vi "Main.vi"() -> ()   [LabVIEW 2023]
uses:
  Application_class/Application.lvclass
  <vilib>/Utility/error.llb/Error Cluster From Error Code.vi
  <vilib>/ErrorRing/Error Ring.xnode
  AFG3022B_class/AFG3022B.lvclass
  CetoniPump_class/CetoniPump.lvclass
  AD2_SDK_class/AD2_SDK.lvclass
  TBS2000Series_class/TBS2000Series.lvclass
  AD2_WFG_SDK_class/AD2TriggerSources.ctl
  AD2_DO_SDK_class/DOTrigger.ctl
  AD2_DO_SDK_class/AD2_DO_SDK.lvclass
  AD2_DO_SDK_class/DOCustomData.ctl
  AD2_DO_SDK_class/DOConfigureCustomData.ctl
  TC0608_class/TC0608.lvclass
  SaveData_class/SaveData.lvclass
  AD2_MSO_SDK_class/AD2TriggerSources.ctl
  AD2_MSO_SDK_class/AD2_MSO_SDK.lvclass
  AD2_MSO_SDK_class/MSORangeCh.ctl
  AD2_MSO_SDK_class/MSOConfig.ctl
panel:
  out "Pump Status":T1(array[cluster])
  in  "Tab Control":T2(tab)=enum."Debug"
  in  "Peltier Controller":bool
  in  "Oscilloscope":bool
  in  "Function Generator":bool
  in  "Cetoni Pump":bool
  in  "Analog Discovery":bool
  in  "Init":bool
  in  "Function Generator":refnum<visa-resource-name>
  in  "Oscilloscope":refnum<visa-resource-name>
  in  "Peltier VISA resource name":refnum<visa-resource-name>
  in  "Device Configuration Folder":string="C:\\Users\\Public\\Documents\\QmixElements\\Projects\\default_project\\Configurations\\sinle"
  in  "Read Peltier":bool
  out "temperature (C)":dbl
  in  "Amplitude Step Number":dbl
  in  "End Amplitude":dbl
  in  "Start Amplitude":dbl
  in  "Frequency Step Size":dbl
  in  "Frequency Step Number":dbl
  in  "Resonance Frequency":dbl
  in  "Voltage Series":bool
  in  "Manual Voltage":bool
  in  "Frequency Series":bool
  in  "Manual Frequency":bool
  in  "Frequency (1000 Hz)":dbl=1000.0
  in  "Amplitude (1 Vpp)":dbl=1.0
  in  "STOP ALL PUMPS!":bool
  in  "GoToLevelSettings":T3
  in  "Go To Level":bool
  in  "Refill":bool
  in  "Index":i32
  in  "Empty":bool
  in  "Read Status":bool
  in  "Configure Syringe":bool
  in  "index configure syringe":i32
  in  "SyringeSettings":T4={"Maximum Piston Stroke (mm)"=100.0, "Inner Diameter (mm)"=12.0}
  in  "Reference Move":bool
  in  "Take Images":bool
  in  "Image  Aquisition":T5={"Minimum Time between frames(s)"=10.0, "Number of Frames"=0} {"Minimum Time between frames(s)" min=0.005}
  in  "Configure MSO":bool
  in  "MSO":T6={"Timing"={"Enable"=TRUE, "Samples In"=100000.0, "Sample Rate"=1250000.0, "Mode"=enum."Single Sample"}, "Trigger"={"Hysteresis"=0.0, "Trigger Level"=0.0, "Trigger Condition"=0, "Trigger Type"=0, "Trigger Channel"=0, "secTimeout"=1.0, "TrigrSrc"=enum."trigrsrcNone"}, "Range Ch1"={"idxChannel"=0, "voltOffset"=0.0, "VoltsRange"=50}, "Range Ch 2"={"idxChannel"=1, "voltOffset"=0.0, "VoltsRange"=50}} {"Range Ch 2"."VoltsRange" items=["High 50V"=50, "Low5V"=5]; "Range Ch1"."VoltsRange" items=["High 50V"=50, "Low5V"=5]; "Trigger"."Trigger Channel" items=["Channel 1"=0, "Channel 2"=1, "Both"=-1]; "Trigger"."Trigger Type" items=["Edge", "Pulse", "Transition"]; "Trigger"."Trigger Condition" items=["Rising", "Falling"]}
  in  "Read MSO":bool
  out "Waveform Graph":waveform(dbl)[](graph)
  in  "Oscilloscope":T9={"Source Main"=2, "Source Probe"=1, "Source Prefocus"=2} {"Source Prefocus" items=["Math", "Channel 1", "Channel 2", "Channel 3", "Channel 4"]; "Source Probe" items=["Math", "Channel 1", "Channel 2", "Channel 3", "Channel 4"]; "Source Main" items=["Math", "Channel 1", "Channel 2", "Channel 3", "Channel 4"]}
  in  "Start Experiment":bool
  out "Temperatur (C)":dbl
  in  "Experiment Settings":T10={"Frequencies (MHz)"=[], "Camera Settings"={"Minimum Time between\n frames(s)"=10.0, "Number of Frames"=0}, "Flowrates (ul/min)"=[], "Voltages (V)"=[]} {"Camera Settings"."Minimum Time between\n frames(s)" min=0.005}
  in  "SaveFolder":path
  out "Oscilloscope Results":T11 {"Probe Current" format="%.2p"; "Phase Angle" format="%.2p"; "Main Freq" format="%.2p"; "Main Volt" format="%.2p"; "Prefocus Freq" format="%.2p"; "Prefocus Volt" format="%.2p"}
  out "LOG":string
  in  "Time To wait":dbl
  in  "Wait":bool
  in  "index":i32
  in  "refill below level":dbl
  in  "Timeout Refill":dbl=20.0 caption="Time Target (s)"
  in  "Check Level and Refill":bool
  in  "Inject Error<Replace Me>":bool
  in  "Trigg AD2":bool
  in  "Configure DO":bool
  in  "?":T12={"DO Trigger"={"secRun(0=Cont)"=0.0, "secWait"=0.0, "cRepeat(0=inf)"=0, "Repeat Trigger"=TRUE, "TrigrSrc"=enum."trigsrcPC"}, "CustomData"=[{"Data"=[FALSE, TRUE, FALSE, FALSE, FALSE, FALSE, FALSE, FALSE, FALSE, FALSE, FALSE, FALSE, FALSE, FALSE, FALSE, FALSE, FALSE, FALSE, FALSE, FALSE, FALSE, FALSE], "Freq"=1000.0, "#Bits"=100, "Enable"=TRUE, "IdleState"=0}, {"Data"=[], "Freq"=0.0, "#Bits"=0, "Enable"=FALSE, "IdleState"=0}, {"Data"=[], "Freq"=0.0, "#Bits"=0, "Enable"=FALSE, "IdleState"=0}, {"Data"=[], "Freq"=0.0, "#Bits"=0, "Enable"=FALSE, "IdleState"=0}, {"Data"=[], "Freq"=0.0, "#Bits"=0, "Enable"=FALSE, "IdleState"=0}, {"Data"=[], "Freq"=0.0, "#Bits"=0, "Enable"=FALSE, "IdleState"=0}, {"Data"=[], "Freq"=0.0, "#Bits"=0, "Enable"=FALSE, "IdleState"=0}, {"Data"=[], "Freq"=0.0, "#Bits"=0, "Enable"=FALSE, "IdleState"=0}, {"Data"=[], "Freq"=0.0, "#Bits"=0, "Enable"=FALSE, "IdleState"=0}, {"Data"=[], "Freq"=0.0, "#Bits"=0, "Enable"=FALSE, "IdleState"=0}, {"Data"=[], "Freq"=0.0, "#Bits"=0, "Enable"=FALSE, "IdleState"=0}, {"Data"=[], "Freq"=0.0, "#Bits"=0, "Enable"=FALSE, "IdleState"=0}, {"Data"=[], "Freq"=0.0, "#Bits"=0, "Enable"=FALSE, "IdleState"=0}, {"Data"=[FALSE, FALSE, FALSE, FALSE, FALSE, FALSE, FALSE, FALSE, FALSE, FALSE, FALSE, FALSE, FALSE, FALSE, FALSE, FALSE, FALSE, FALSE, FALSE, FALSE, FALSE, FALSE, FALSE], "Freq"=0.0, "#Bits"=0, "Enable"=FALSE, "IdleState"=0}, {"Data"=[FALSE, FALSE, FALSE, FALSE, FALSE, FALSE, FALSE, FALSE, FALSE, FALSE, FALSE, FALSE, FALSE, FALSE, FALSE, FALSE, FALSE, FALSE, FALSE, FALSE, FALSE, FALSE, FALSE], "Freq"=0.0, "#Bits"=0, "Enable"=FALSE, "IdleState"=0}]}
  in  "ABORT":bool
  out "Status":string="Program Started\nPlease connect to instruments"
  out "error out":errorcluster
  in  "Exit":bool
  # "Include connection of Pump, Camera and Multimeter as well. Have some feedback (LED) if connected."
  # "Select Instruments to Initialize"
  # "FREQUENCY"
  # "VOLTAGE"
  # "There needs to be some build-in control to reverse the pump (refilling it and mixing the particles at the same time) \nafter each completed Frequency Series"
  # "Makse sure to set minimim time large enough, otherwise camera will ignore triggers and we skip frames\nSince we are not running with SDK we cannot know if Images are taken or not"
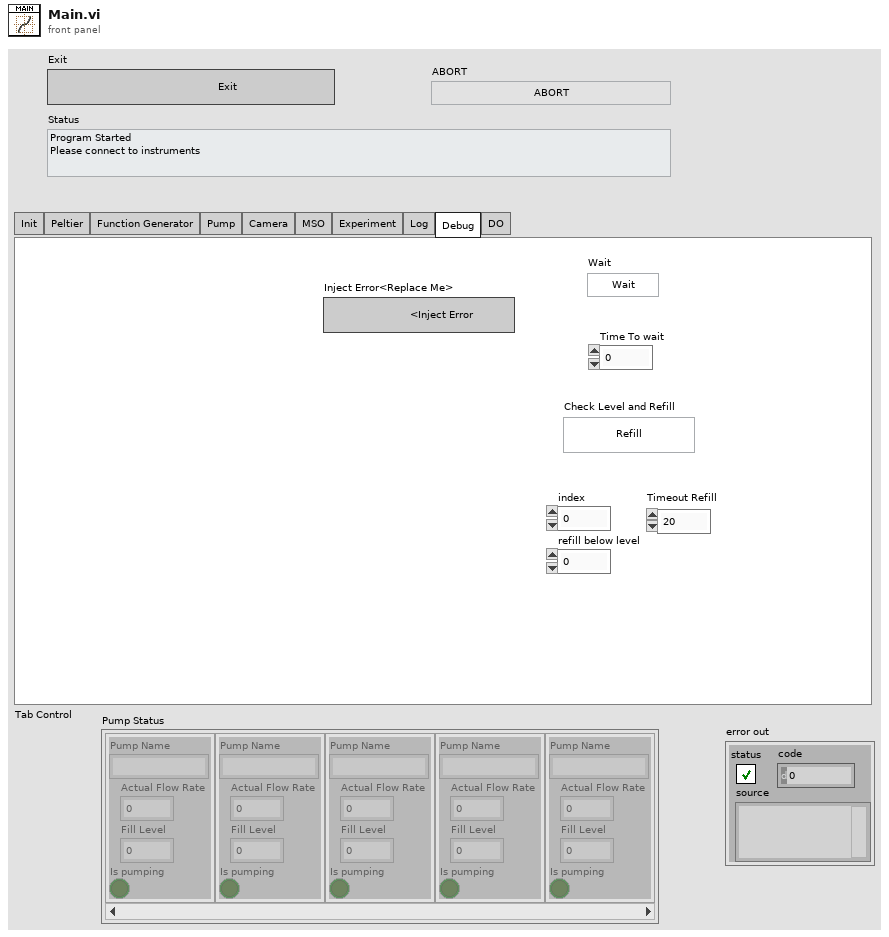
[diagram p1: front panel]
types:
  T1 = cluster{"Pump Name":string, "Actual Flow Rate":dbl, "Fill Level":dbl, "Is pumping":bool}[]
  T2 = enum32{"Init", "Peltier", "Function Generator", "Pump", "Camera", "MSO", "Experiment", "Log", "Debug", "DO"}
  T3 = cluster{"index":i32, "Level(ml)":dbl, "Flow":dbl}
  T4 = cluster{"Maximum Piston Stroke (mm)":dbl, "Inner Diameter (mm)":dbl}
  T5 = cluster{"Minimum Time between frames(s)":dbl, "Number of Frames":i32}
  T6 = typedef "AD2_MSO_SDK.lvclass/MSOConfig.ctl" = cluster{"Timing":cluster{"Enable":bool, "Samples In":dbl, "Sample Rate":dbl, "Mode":enum16{"Single Sample", "Scanshift", "Multiple Samples", "Scan Screen"}}, "Trigger":cluster{"Hysteresis":dbl, "Trigger Level":dbl, "Trigger Condition":i32, "Trigger Type":i32, "Trigger Channel":i32, "secTimeout":dbl, "TrigrSrc":T7}, "Range Ch1":T8, "Range Ch 2":T8}
  T7 = typedef "AD2_MSO_SDK.lvclass/AD2TriggerSources.ctl" = enum8{"trigrsrcNone", "trigsrcPC", "trigsrcDetectorAnalogIn", "trigsrcDetectorDigitalIn", "trigsrcAnalogIn", "trigsrcDigitalIn", "trigsrcDigitalOut", "trigsrcAnalogOut1", "trigsrcAnalogOut2", "trigsrcAnalogOut3", "trigsrcAnalogOut4", "trigsrcExternal1", "trigsrcExternal2", "trigsrcExternal3", "trigsrcExternal4", ""}
  T8 = typedef "AD2_MSO_SDK.lvclass/MSORangeCh.ctl" = cluster{"idxChannel":i32, "voltOffset":dbl, "VoltsRange":u16}
  T9 = cluster{"Source Main":i32, "Source Probe":i32, "Source Prefocus":i32}
  T10 = cluster{"Frequencies (MHz)":dbl[], "Camera Settings":cluster{"Minimum Time between\n frames(s)":dbl, "Number of Frames":i32}, "Flowrates (ul/min)":dbl[], "Voltages (V)":dbl[]}
  T11 = cluster{"Prefocus":cluster{"Initial X":dbl, "X Increment":dbl, "Waveform Array":dbl[]}, "Prefocus Volt":dbl, "Prefocus Freq":dbl, "Main":cluster{"Initial X":dbl, "X Increment":dbl, "Waveform Array":dbl[]}, "Main Volt":dbl, "Main Freq":dbl, "Phase Angle":dbl, "Probe Current":dbl, "Power (Watt)":dbl}
  T12 = typedef "DOConfigureCustomData.ctl" = cluster{"DO Trigger":T13, "CustomData":T15}
  T13 = typedef "AD2_DO_SDK.lvclass/DOTrigger.ctl" = cluster{"secRun(0=Cont)":dbl, "secWait":dbl, "cRepeat(0=inf)":i32, "Repeat Trigger":bool, "TrigrSrc":T14}
  T14 = typedef "AD2_SDK.lvclass/AD2TriggerSources.ctl" = enum8{"trigrsrcNone", "trigsrcPC", "trigsrcDetectorAnalogIn", "trigsrcDetectorDigitalIn", "trigsrcAnalogIn", "trigsrcDigitalIn", "trigsrcDigitalOut", "trigsrcAnalogOut1", "trigsrcAnalogOut2", "trigsrcAnalogOut3", "trigsrcAnalogOut4", "trigsrcExternal1", "trigsrcExternal2", "trigsrcExternal3", "trigsrcExternal4", ""}
  T15 = typedef "AD2_DO_SDK.lvclass/DOCustomData.ctl" = cluster{"Data":bool[], "Freq":dbl, "#Bits":u32, "Enable":bool, "IdleState":u16}[]
  T16 = cluster{"Minimum Time between frames":dbl, "Number of Frames":i32}
  T17 = cluster{"Pump Handle":i64, "Pump Name":string, "Maximum Volume":dbl, "Maximum Flow Rate":dbl, "Flow Rate":dbl, "Target Level":dbl, "Valve Handle":i64, "Has Valve?":bool, "Actual valve position":i32}[]
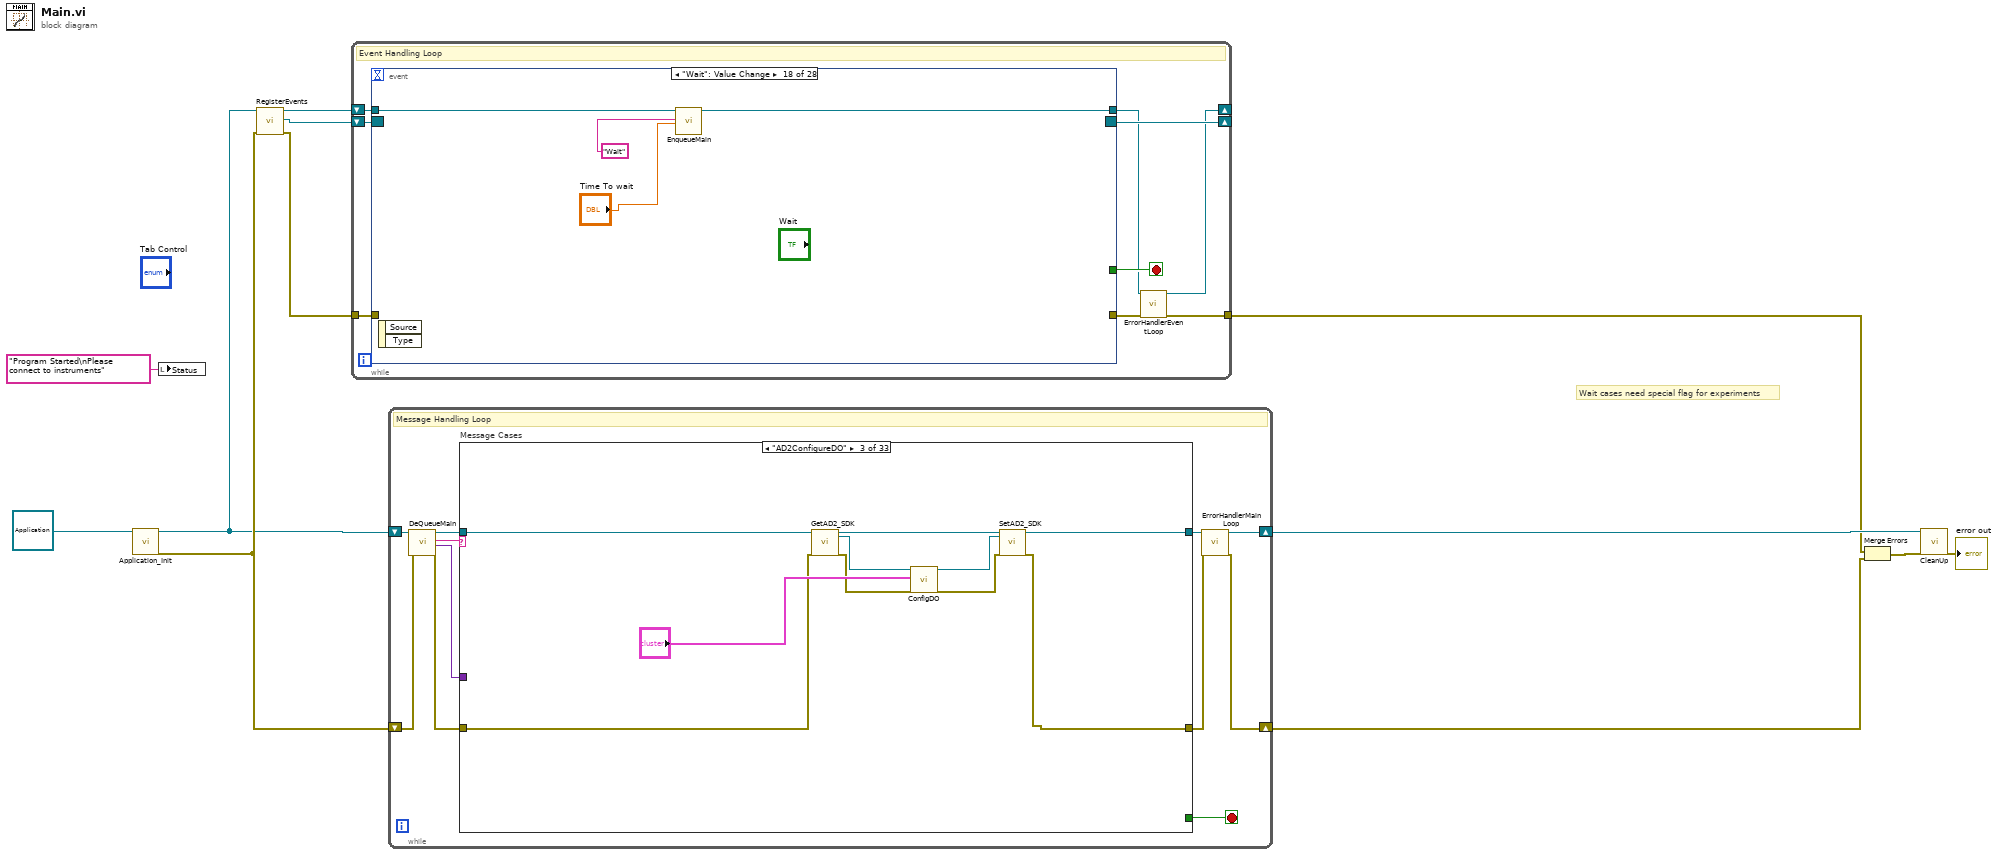
[diagram p0: block diagram]
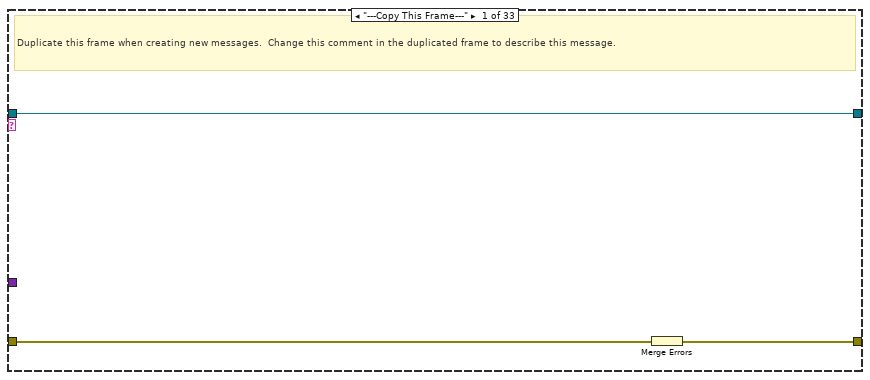
[diagram p2: hidden frame]
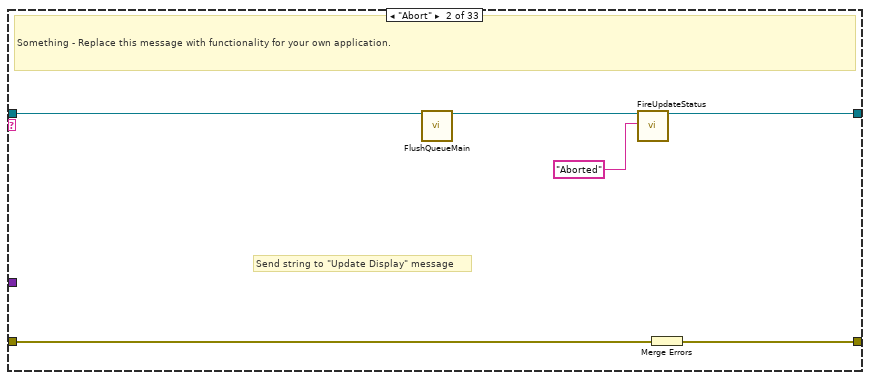
[diagram p3: hidden frame]
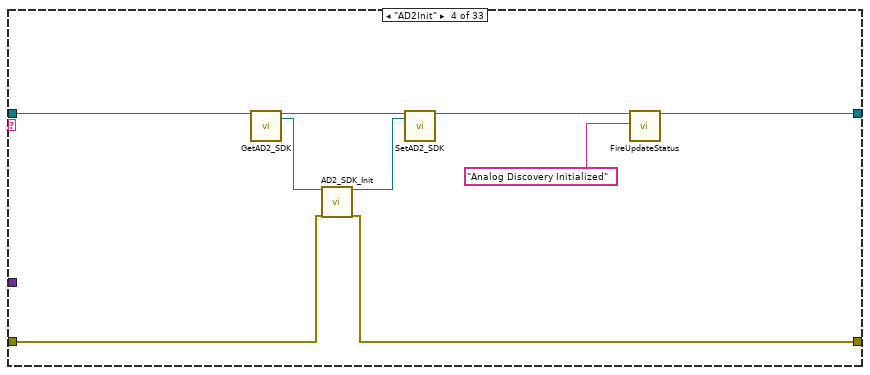
[diagram p4: hidden frame]
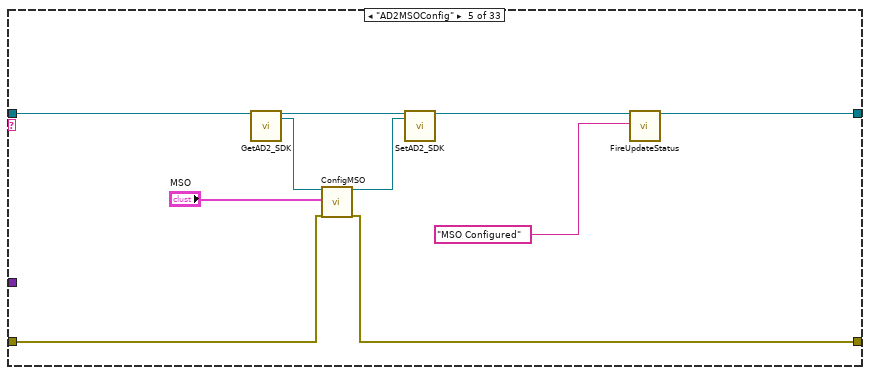
[diagram p5: hidden frame]
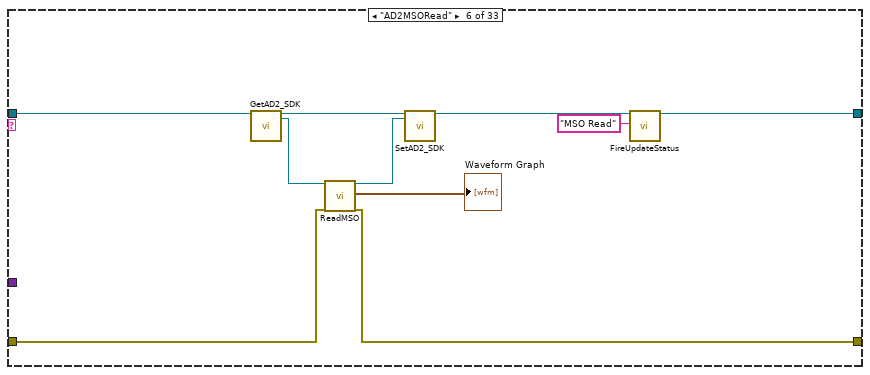
[diagram p6: hidden frame]
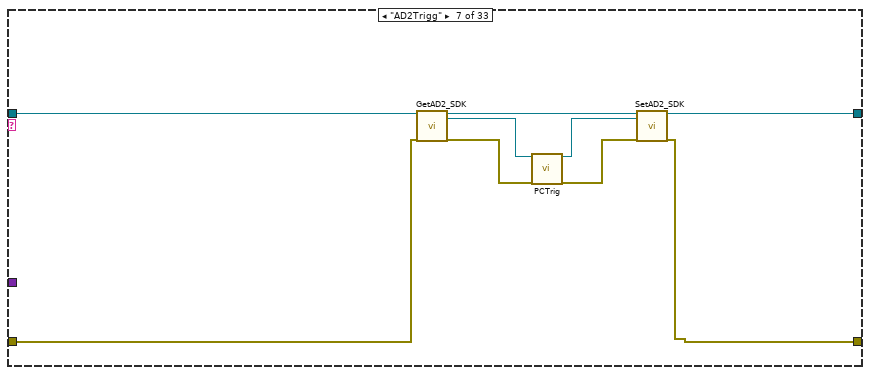
[diagram p7: hidden frame]
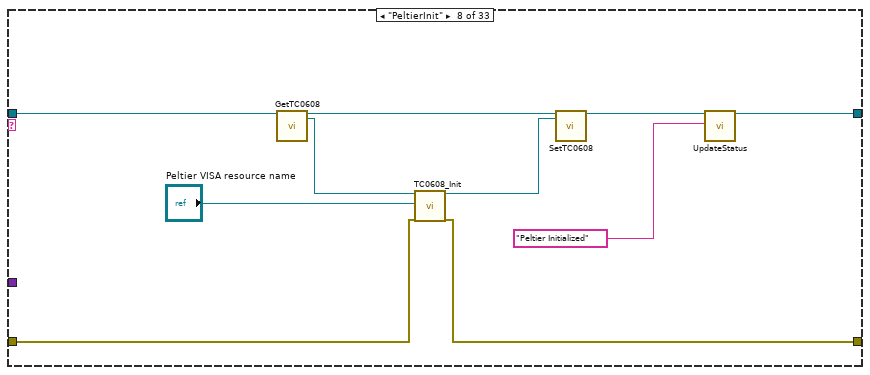
[diagram p8: hidden frame]
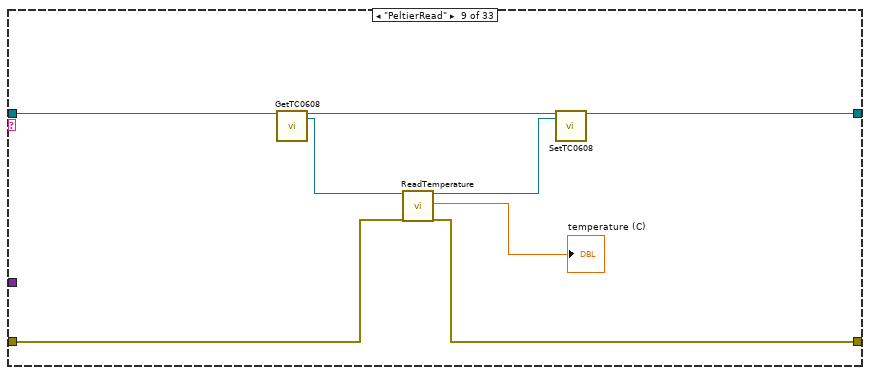
[diagram p9: hidden frame]
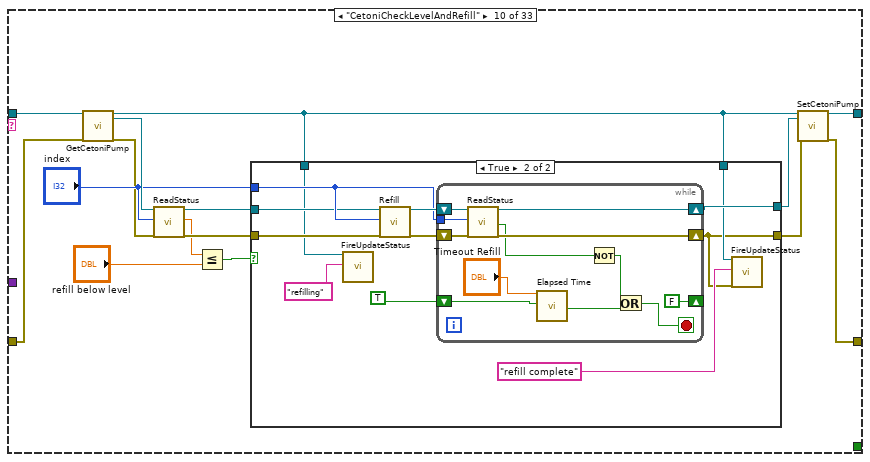
[diagram p10: hidden frame]
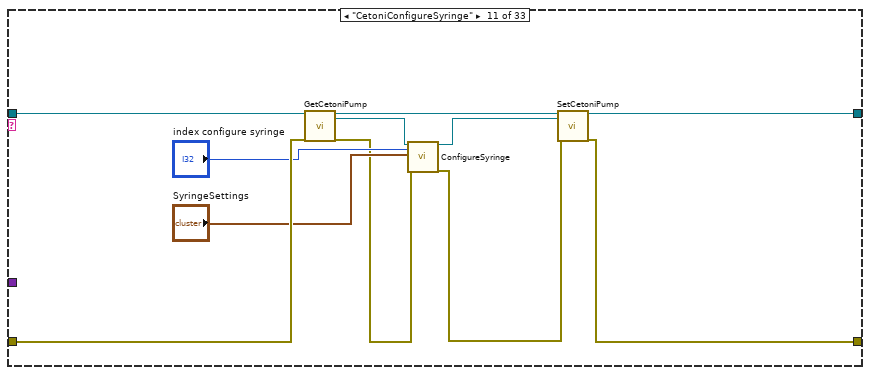
[diagram p12: hidden frame]
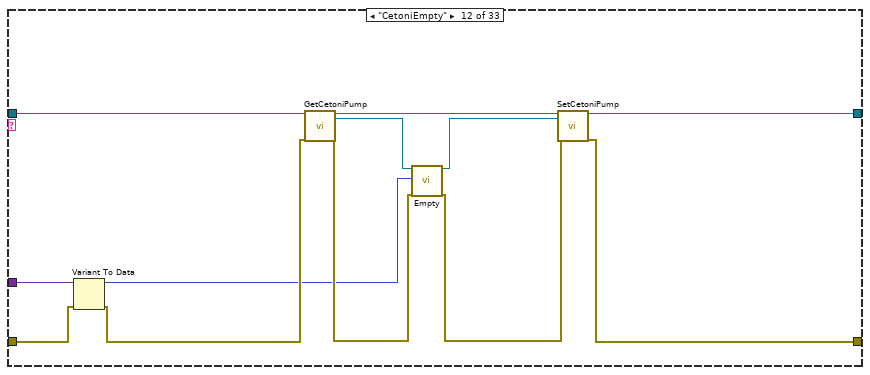
[diagram p13: hidden frame]
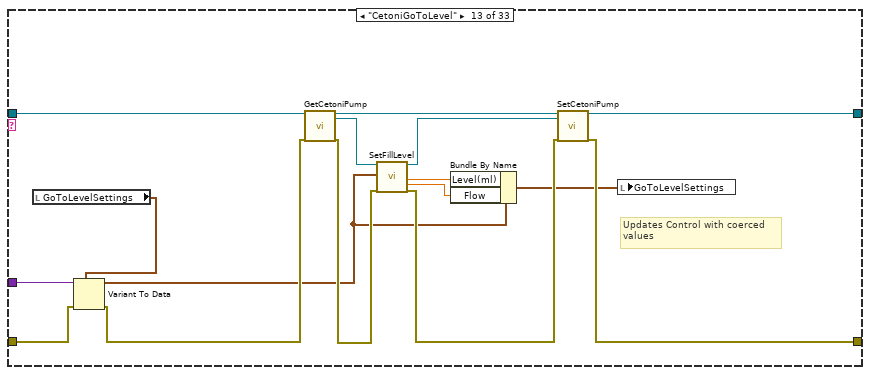
[diagram p14: hidden frame]
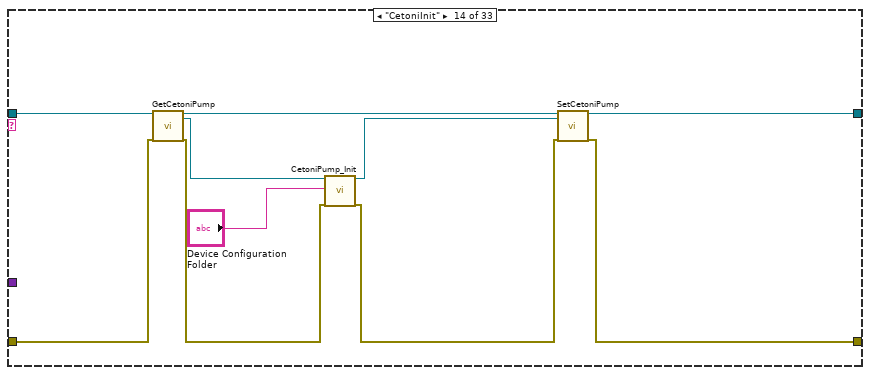
[diagram p15: hidden frame]
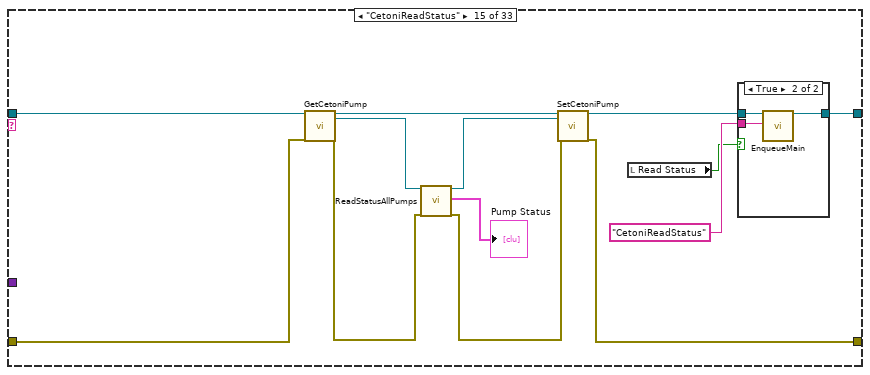
[diagram p16: hidden frame]
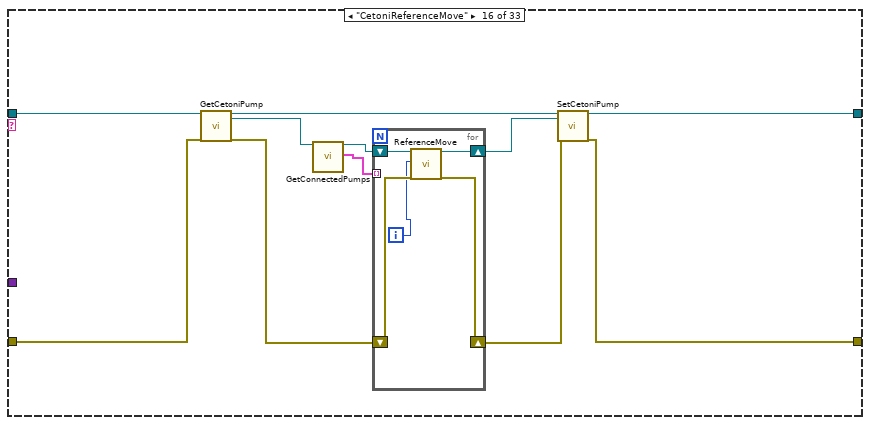
[diagram p18: hidden frame]
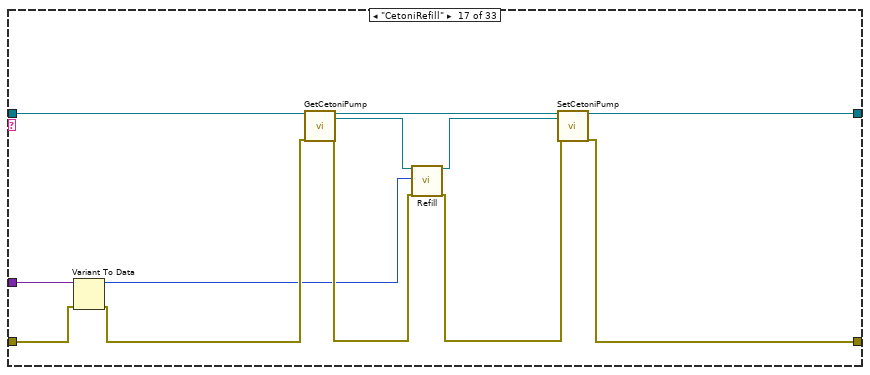
[diagram p19: hidden frame]
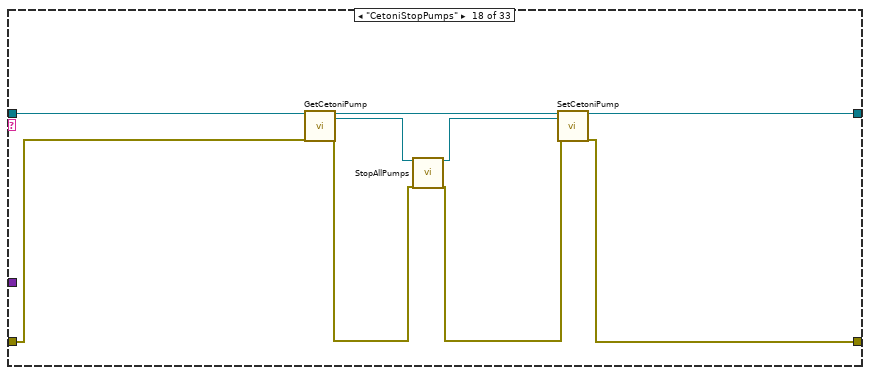
[diagram p20: hidden frame]
diagram:
  # "Wait cases need special flag for experiments"
  n1 = call "Application_Init.vi"("object in"=refnum<class "Application.lvclass"> refnum ("Application")) -> ("object out"=w2:refnum<class "Application.lvclass">, "error out"=w8:errorcluster)  [unwired: 17 in]
  n2 = local write "Status"("Program Started\nPlease connect to instruments" ("Status")) -> ()
  n3 = call-dynamic "RegisterEvents.vi"("object in"=w2, "error in (no error)"=w8) -> ("object out"=w10:refnum<class "Application.lvclass">, "Event Registration Refnum"=w11:refnum<event-registration>, "error out"=w9:errorcluster)  [unwired: 15 in]
  n4 = while {
    shift-right: [w20] -> _
    shift-left: w11 -> [w21]
    tunnel: [w15] -> w5
    shift-right: [w13] -> _
    shift-left: w10 -> [w18]
    tunnel: w9 -> [w17]
    stop <- w19 stop-if-true
    # "Event Handling Loop"
    n5 = event shown="[17] \"Wait\": Value Change" {
      selector: w21 -> [_ _ _ _ _ _ _ _ _ _ _ _ _ _ _ _ _ _ _ _ _ _ _ _ _ _ _ _]
      dyn-events: [_ _ _ _ _ _ _ _ _ _ _ _ _ _ _ _ _ _ _ _ _ _ _ _ _ _ _ _] -> w20
      timeout: _ -> [_ _ _ _ _ _ _ _ _ _ _ _ _ _ _ _ _ _ _ _ _ _ _ _ _ _ _ _]
      tunnel: [_ _ _ _ _ _ _ _ _ _ _ _ _ _ _ _ _ _ _ _ _ _ _ _ _ _ TRUE ("Discard?") _] -> w19
      tunnel: [w22 w28 w36 w42 w47 _ _ _ _ _ w129 _ _ _ _ _ _ _ w159 w166 w177 w183 _ _ w195 w200 _ w207] -> w16
      tunnel: w18 -> [w27 w33 w39 w41 w48 w50 w87 w99 w110 w120 w133 w136 w139 w142 w145 w149 w151 w156 w160 w167 w178 w184 w189 w192 w196 w201 w204 w210]
      tunnel: [w26 w32 w38 w40 w48 w51 w87 w99 w110 w120 w132 w135 w138 w141 w144 w148 w152 w155 w161 w168 w179 w185 w188 w191 w197 w202 w204 w210] -> w14
      tunnel: w17 -> [w23 w29 w35 w43 w47 _ _ _ _ _ w130 _ _ _ _ _ _ _ w158 w165 w176 w182 _ _ w194 w199 _ w208]
      event "Exit": Value Change {
        n6 = event-data() -> ()  [unwired: 1 in, 1 out]
        n7 = call-dynamic "EnqueueMain.vi"("object in"=w27, "Message"="Exit", "error in (no error)"=w23, "Priority Message? (F)"=TRUE) -> ("object out"=w26:refnum<class "Application.lvclass">, "error out"=w22:errorcluster)  [unwired: 14 in]
      }
      event "ABORT": Value Change {
        n8 = event-data() -> ()  [unwired: 1 in, 1 out]
        n9 = call-dynamic "EnqueueMain.vi"("object in"=w33, "Message"="Abort", "error in (no error)"=w29, "Priority Message? (F)"=TRUE) -> ("object out"=w32:refnum<class "Application.lvclass">, "error out"=w28:errorcluster)  [unwired: 14 in]
      }
      event "Inject Error<Replace Me>": Value Change {
        # "#CodeNeeded - Send the appropriate message for this user interface event."
        n10 = event-data() -> ()  [unwired: 1 in, 1 out]
        n11 = call-dynamic "EnqueueMain.vi"("object in"=w39, "Message"="InjectError", "Message Data"=errorcluster {"status"=TRUE, "code"=-8000, "source"="Injected Error"} ("error in (no error)"), "error in (no error)"=w35) -> ("object out"=w38:refnum<class "Application.lvclass">, "error out"=w36:errorcluster)  [unwired: 14 in]
      }
      event Panel Close? {
        # "Send the 'Confirm Quit' message if the user closes the panel of the VI. Discard the event so the 'Confirm Quit' message has a chance to run."
        n12 = event-data() -> ()  [unwired: 1 in, 1 out]
        n13 = call-dynamic "EnqueueMain.vi"("object in"=w41, "Message"="Confirm Quit", "error in (no error)"=w43, "Priority Message? (F)"=TRUE) -> ("object out"=w40:refnum<class "Application.lvclass">, "error out"=w42:errorcluster)  [unwired: 14 in]
        n14 = event-data("Discard?"=TRUE) -> ()  [unwired: 1 in, 1 out]
      }
      event Application Instance Close {
        # "#CodeRecommended - When a project closes, all VIs within that project are aborted and leave memory. However, any code placed in this event frame is guaranteed to run to completion, so add any cleanup code that absolutely must happen here."
        n15 = event-data() -> ()  [unwired: 1 in, 1 out]
      }
      event "Init": Value Change {
        n16 = event-data() -> ()  [unwired: 1 in, 2 out]
        n17 = case shown="False" "Function Generator" {
          tunnel: w50 -> [w81 w84]
          tunnel: [w81 w83] -> w64
          tunnel: "FuncInit" ("Message") -> [_ w82]
          frame False {
          }
          frame True {
            n18 = call-dynamic "EnqueueMain.vi"("object in"=w84, "Message"=w82) -> ("object out"=w83:refnum<class "Application.lvclass">)  [unwired: 16 in, 1 out]
          }
        }
        n19 = case shown="False" "Cetoni Pump" {
          tunnel: w64 -> [w77 w80]
          tunnel: "CetoniInit" ("Message") -> [_ w79]
          tunnel: [w77 w78] -> w61
          frame False {
          }
          frame True {
            n20 = call-dynamic "EnqueueMain.vi"("object in"=w80, "Message"=w79) -> ("object out"=w78:refnum<class "Application.lvclass">)  [unwired: 16 in, 1 out]
          }
        }
        n21 = case shown="False" "Analog Discovery" {
          tunnel: w61 -> [w73 w76]
          tunnel: "AD2Init" ("Message") -> [_ w75]
          tunnel: [w73 w74] -> w57
          frame False {
          }
          frame True {
            n22 = call-dynamic "EnqueueMain.vi"("object in"=w76, "Message"=w75) -> ("object out"=w74:refnum<class "Application.lvclass">)  [unwired: 16 in, 1 out]
          }
        }
        n23 = case shown="True" "Oscilloscope" {
          tunnel: w57 -> [w69 w72]
          tunnel: "OscilloscopeInit" ("Message") -> [_ w71]
          tunnel: [w69 w70] -> w54
          frame False {
          }
          frame True {
            n24 = call-dynamic "EnqueueMain.vi"("object in"=w72, "Message"=w71) -> ("object out"=w70:refnum<class "Application.lvclass">)  [unwired: 16 in, 1 out]
          }
        }
        n25 = case shown="True" "Peltier Controller" {
          tunnel: w54 -> [w65 w68]
          tunnel: "PeltierInit" ("Message") -> [_ w67]
          tunnel: [w65 w66] -> w51
          frame False {
          }
          frame True {
            n26 = call-dynamic "EnqueueMain.vi"("object in"=w68, "Message"=w67) -> ("object out"=w66:refnum<class "Application.lvclass">)  [unwired: 16 in, 1 out]
          }
        }
      }
      event "Manual Frequency": Value Change {
        n27 = event-data() -> ()  [unwired: 1 in, 2 out]
        n28 = call-dynamic "EnqueueMain.vi"("object in"=w87, "Message"="ChangeFrequency", "Message Data"="Frequency (1000 Hz)") -> ()  [unwired: 15 in, 2 out]
      }
      event "Frequency Series": Value Change {
        n29 = event-data() -> ()  [unwired: 1 in, 2 out]
        n30 = Multiply(x="Frequency Step Number", y="Frequency Step Size") -> (x*y=w96:dbl)
        n31 = Multiply(x="Frequency Step Number", y=2.0) -> (x*y=w90:dbl)
        n32 = Subtract(x="Resonance Frequency", y=w96) -> (x-y=w95:dbl)
        n33 = Add(x=w90, y=1.0) -> (x+y=w88:dbl)
        n34 = for {
          N: w88 -> [_]
          tunnel: w95 -> [w104]
          tunnel: "Frequency Step Size" -> [w102]
          tunnel: [w100] -> w93 mode=indexing
          i -> [w101]
          n35 = Multiply(x=w102, y=w101) -> (x*y=w103:dbl)
          n36 = Add(x=w104, y=w103) -> (x+y=w100:dbl)
        }
        n37 = for {
          tunnel: w99 -> [w107]
          tunnel: "ChangeFrequency" ("Message") -> [w106]
          tunnel: w93 -> [w105] mode=indexing
          n38 = call-dynamic "EnqueueMain.vi"("object in"=w107, "Message"=w106, "Message Data"=w105) -> ()  [unwired: 15 in, 2 out]
        }
      }
      event "Manual Voltage": Value Change {
        n39 = event-data() -> ()  [unwired: 1 in, 2 out]
        n40 = call-dynamic "EnqueueMain.vi"("object in"=w110, "Message"="ChangeVoltage", "Message Data"="Amplitude (1 Vpp)") -> ()  [unwired: 15 in, 2 out]
      }
      event "Voltage Series": Value Change {
        n41 = event-data() -> ()  [unwired: 1 in, 2 out]
        n42 = Subtract(x="End Amplitude", y="Start Amplitude") -> (x-y=w117:dbl)
        n43 = Divide(x=w117, y="Amplitude Step Number") -> (x/y=w116:dbl)
        n44 = Add(x="Amplitude Step Number", y=1.0) -> (x+y=w111:dbl)
        n45 = for {
          N: w111 -> [_]
          tunnel: w116 -> [w124]
          tunnel: "Start Amplitude" -> [w122]
          tunnel: [w121] -> w114 mode=indexing
          i -> [w125]
          n46 = Multiply(x=w124, y=w125) -> (x*y=w123:dbl)
          n47 = Add(x=w122, y=w123) -> (x+y=w121:dbl)
        }
        n48 = for {
          tunnel: w120 -> [w128]
          tunnel: "ChangeVoltage" ("Message") -> [w127]
          tunnel: w114 -> [w126] mode=indexing
          n49 = call-dynamic "EnqueueMain.vi"("object in"=w128, "Message"=w127, "Message Data"=w126) -> ()  [unwired: 15 in, 2 out]
        }
      }
      event "Read Peltier": Value Change {
        n50 = event-data() -> ()  [unwired: 1 in, 2 out]
        n51 = call-dynamic "EnqueueMain.vi"("object in"=w133, "Message"="PeltierRead", "error in (no error)"=w130) -> ("object out"=w132:refnum<class "Application.lvclass">, "error out"=w129:errorcluster)  [unwired: 15 in]
      }
      event "Configure DO": Value Change {
        n52 = event-data() -> ()  [unwired: 1 in, 2 out]
        n53 = call-dynamic "EnqueueMain.vi"("object in"=w136, "Message"="AD2ConfigureDO") -> ("object out"=w135:refnum<class "Application.lvclass">)  [unwired: 16 in, 1 out]
      }
      event "Configure MSO": Value Change {
        n54 = event-data() -> ()  [unwired: 1 in, 2 out]
        n55 = call-dynamic "EnqueueMain.vi"("object in"=w139, "Message"="AD2MSOConfig") -> ("object out"=w138:refnum<class "Application.lvclass">)  [unwired: 16 in, 1 out]
      }
      event "Read MSO": Value Change {
        n56 = event-data() -> ()  [unwired: 1 in, 2 out]
        n57 = call-dynamic "EnqueueMain.vi"("object in"=w142, "Message"="AD2MSORead") -> ("object out"=w141:refnum<class "Application.lvclass">)  [unwired: 16 in, 1 out]
      }
      event "Trigg AD2": Value Change {
        n58 = event-data() -> ()  [unwired: 1 in, 2 out]
        n59 = call-dynamic "EnqueueMain.vi"("object in"=w145, "Message"="AD2Trigg") -> ("object out"=w144:refnum<class "Application.lvclass">)  [unwired: 16 in, 1 out]
      }
      event "Take Images": Value Change {
        n60 = event-data() -> ()  [unwired: 1 in, 2 out]
        n61 = call-dynamic "EnqueueMain.vi"("object in"=w149, "Message"="TakeNImages", "Message Data"="Image  Aquisition") -> ("object out"=w148:refnum<class "Application.lvclass">)  [unwired: 15 in, 1 out]
      }
      event "Start Experiment": Value Change {
        # "I made a Subvi to fit screen"
        n62 = event-data() -> ()  [unwired: 1 in, 2 out]
        n63 = call-dynamic "BuildExperiment.vi"("object in"=w151, "Experiment Settings"="Experiment Settings") -> ("object out"=w152:refnum<class "Application.lvclass">)  [unwired: 16 in, 1 out]
      }
      event "Wait": Value Change {
        n64 = event-data() -> ()  [unwired: 1 in, 2 out]
        n65 = call-dynamic "EnqueueMain.vi"("object in"=w156, "Message"="Wait", "Message Data"="Time To wait") -> ("object out"=w155:refnum<class "Application.lvclass">)  [unwired: 15 in, 1 out]
      }
      event "Go To Level": Value Change {
        n66 = event-data() -> ()  [unwired: 1 in, 2 out]
        n67 = call-dynamic "EnqueueMain.vi"("object in"=w160, "Message"="CetoniGoToLevel", "Message Data"="GoToLevelSettings", "error in (no error)"=w158) -> ("object out"=w161:refnum<class "Application.lvclass">, "error out"=w159:errorcluster)  [unwired: 14 in]
      }
      event "Reference Move": Value Change {
        n68 = event-data() -> ()  [unwired: 1 in, 2 out]
        n69 = Two Button Dialog(message="The pumps will perform a reference move. Please remove all syringes!!!!! ") -> (T button?=w164:bool)  [unwired: 2 in]
        n70 = case shown="True" w164 {
          tunnel: [w169 w174] -> w168
          tunnel: w167 -> [w169 w173]
          tunnel: [w170 w172] -> w166
          tunnel: w165 -> [w170 w171]
          frame False {
          }
          frame True {
            n71 = call-dynamic "EnqueueMain.vi"("object in"=w173, "Message"="CetoniReferenceMove", "error in (no error)"=w171) -> ("object out"=w174:refnum<class "Application.lvclass">, "error out"=w172:errorcluster)  [unwired: 15 in]
          }
        }
      }
      event "Configure Syringe": Value Change {
        n72 = event-data() -> ()  [unwired: 1 in, 2 out]
        n73 = call-dynamic "EnqueueMain.vi"("object in"=w178, "Message"="CetoniConfigureSyringe", "error in (no error)"=w176) -> ("object out"=w179:refnum<class "Application.lvclass">, "error out"=w177:errorcluster)  [unwired: 15 in]
      }
      event "Refill": Value Change {
        n74 = event-data() -> ()  [unwired: 1 in, 2 out]
        n75 = call-dynamic "EnqueueMain.vi"("object in"=w184, "Message"="CetoniRefill", "Message Data"="Index", "error in (no error)"=w182) -> ("object out"=w185:refnum<class "Application.lvclass">, "error out"=w183:errorcluster)  [unwired: 14 in]
      }
      event "Check Level and Refill": Value Change {
        n76 = event-data() -> ()  [unwired: 1 in, 2 out]
        n77 = call-dynamic "EnqueueMain.vi"("object in"=w189, "Message"="CetoniCheckLevelAndRefill") -> ("object out"=w188:refnum<class "Application.lvclass">)  [unwired: 16 in, 1 out]
      }
      event "STOP ALL PUMPS!": Value Change {
        n78 = event-data() -> ()  [unwired: 1 in, 2 out]
        n79 = call-dynamic "EnqueueMain.vi"("object in"=w192, "Message"="CetoniStopPumps") -> ("object out"=w191:refnum<class "Application.lvclass">)  [unwired: 16 in, 1 out]
      }
      event "Empty": Value Change {
        n80 = event-data() -> ()  [unwired: 1 in, 2 out]
        n81 = local read "Index"() -> (w193:i32)
        n82 = call-dynamic "EnqueueMain.vi"("object in"=w196, "Message"="CetoniEmpty", "Message Data"=w193, "error in (no error)"=w194) -> ("object out"=w197:refnum<class "Application.lvclass">, "error out"=w195:errorcluster)  [unwired: 14 in]
      }
      event "Read Status": Value Change {
        n83 = event-data() -> ()  [unwired: 1 in, 2 out]
        n84 = call-dynamic "EnqueueMain.vi"("object in"=w201, "Message"="CetoniReadStatus", "error in (no error)"=w199) -> ("object out"=w202:refnum<class "Application.lvclass">, "error out"=w200:errorcluster)  [unwired: 15 in]
      }
      event User Event {
        (unwired) "\"Exit\" button pressed" ("VI Stopped")
        # "The Message Handling Loop processed an \"Exit\" message, which fired this event to stop the Event Handling Loop."
        n85 = event-data() -> ()  [unwired: 1 in, 1 out]
      }
      event User Event {
        n86 = event-data() -> ("Message"=w209:string, "Message Data"=w206:variant)  [unwired: 1 in]
        n87 = case shown="\"UpdateStatus\"" w209 {
          tunnel: w208 -> [w214 w223]
          tunnel: [w214 w223] -> w207
          tunnel: w206 -> [w213 _]
          frame "UpdateStatus" {
            # "I have disabled the log, it might slow down the program\nwhen it becomes to large"
            n88 = Variant To Data(type="" ("Status"), Variant=w213) -> (data=w211:string)  [unwired: 1 in, 1 out]
            "Status" <- w211
            n89 = disable-structure shown="Disabled" {
              disable-tunnel: w211 -> [w218 _]
              frame Disabled {
                n90 = Get Date/Time In Seconds() -> (seconds since 1Jan1904=w222:timestamp)
                n91 = Get Date/Time String(seconds (now)=w222) -> (time string=w219:string)  [unwired: 2 in, 1 out]
                n92 = feedback #1("" ("string")) -> (w215:string)
                n93 = Concatenate Strings(w215, "\r", w219, "\t", w218) -> (w217:string)
                "LOG" <- w217
                n94 = feedback-in #1(w217) -> ()
              }
              frame Enabled {
              }
            }
          }
          frame Default {
          }
        }
      }
    }
    n95 = call-dynamic "ErrorHandlerEventLoop.vi"("object in"=w14, "error in (no error)"=w16) -> ("object out"=w13:refnum<class "Application.lvclass">, "error out"=w15:errorcluster)  [unwired: 16 in]
  }
  n96 = while {
    shift-right: [w227] -> w7
    shift-left: w2 -> [w233]
    shift-right: [w228] -> w6
    shift-left: w8 -> [w224]
    stop <- w234 stop-if-true
    # "Message Handling Loop"
    n97 = call-dynamic "DeQueueMain.vi"("object in"=w233, "error in (no error)"=w224) -> ("object out"=w232:refnum<class "Application.lvclass">, "Message"=w231:string, "Message Data"=w230:variant, "error out"=w225:errorcluster)  [unwired: 14 in]
    n98 = case "Message Cases" shown="\"AD2ConfigureDO\"" w231 {
      selector: w231 -> [_ _ _ _ _ _ _ _ _ _ _ _ _ _ _ _ _ _ _ _ _ _ _ _ _ _ _ _ _ _ _ _ w601]
      tunnel: w225 -> [w237 w242 w244 w258 w268 w277 w287 w294 w304 w321 w357 w367 w378 w397 w409 w423 w438 w449 w461 w477 w488 w490 w495 w512 w517 w529 w532 w534 w554 w560 w565 w597 _]
      tunnel: [w236 w243 w245 w259 w269 w276 w288 w295 w303 w322 w359 w371 w387 w396 w411 w425 w442 w451 w462 w478 w483 w491 w496 w512 w522 w528 w532 w534 w542 w561 w566 w593 w602] -> w229
      tunnel: [_ _ _ _ _ _ _ _ _ _ _ _ _ _ _ _ _ _ _ _ _ TRUE _ _ _ _ _ _ _ _ _ _ _] -> w234
      tunnel: w230 -> [_ _ _ _ _ _ _ _ _ _ _ w369 w380 _ _ _ w440 _ w463 w479 w487 _ _ _ w520 _ _ _ w540 _ w568 w599 _]
      tunnel: w232 -> [w235 w241 w253 w262 w272 w282 w291 w297 w307 w324 w361 w373 w389 w399 w412 w427 w444 w453 w464 w480 w482 w492 w500 w507 w521 w526 w531 w533 w558 w559 w572 w595 w600]
      tunnel: [w235 w239 w251 w255 w264 w275 w289 w293 w308 w323 w360 w372 w388 w398 w401 w426 w443 w452 w459 w475 w482 w493 w501 w508 w521 w525 w531 w533 w545 w559 w573 w590 w600] -> w226
      frame "---Copy This Frame---" {
        # "Duplicate this frame when creating new messages.  Change this comment in the duplicated frame to describe this message."
        n99 = Merge Errors(w237) -> (w236:errorcluster)
      }
      frame "Abort" {
        # "Send string to \"Update Display\" message"
        # "Something - Replace this message with functionality for your own application."
        n100 = call-dynamic "FlushQueueMain.vi"("object in"=w241) -> ("object out"=w240:refnum<class "Application.lvclass">)  [unwired: 16 in, 2 out]
        n101 = call-dynamic "FireUpdateStatus.vi"("object in"=w240, "Status"="Aborted") -> ("object out"=w239:refnum<class "Application.lvclass">)  [unwired: 16 in, 1 out]
        n102 = Merge Errors(w242) -> (w243:errorcluster)
      }
      frame "AD2ConfigureDO" {
        n103 = call-dynamic "GetAD2_SDK.vi"("object in"=w253, "error in (no error)"=w244) -> ("object out"=w252:refnum<class "Application.lvclass">, "AD2_SDK"=w249:refnum<class "AD2_SDK.lvclass">, "error out"=w248:errorcluster)  [unwired: 15 in]
        n104 = call-dynamic "ConfigDO.vi"("object in"=w249, 2:"?", "error in (no error)"=w248) -> ("object out"=w247:refnum<class "AD2_SDK.lvclass">, "error out"=w246:errorcluster)  [unwired: 15 in]
        n105 = call-dynamic "SetAD2_SDK.vi"("object in"=w252, "AD2_SDK"=w247, "error in (no error)"=w246) -> ("object out"=w251:refnum<class "Application.lvclass">, "error out"=w245:errorcluster)  [unwired: 15 in]
      }
      frame "AD2Init" {
        n106 = call-dynamic "GetAD2_SDK.vi"("object in"=w262) -> ("object out"=w261:refnum<class "Application.lvclass">, "AD2_SDK"=w257:refnum<class "AD2_SDK.lvclass">)  [unwired: 16 in, 1 out]
        n107 = call "AD2_SDK_Init.vi"("object in"=w257, "error in (no error)"=w258) -> ("object out"=w256:refnum<class "AD2_SDK.lvclass">, "error out"=w259:errorcluster)  [unwired: 16 in]
        n108 = call-dynamic "SetAD2_SDK.vi"("object in"=w261, "AD2_SDK"=w256) -> ("object out"=w260:refnum<class "Application.lvclass">)  [unwired: 16 in, 1 out]
        n109 = call-dynamic "FireUpdateStatus.vi"("object in"=w260, "Status"="Analog Discovery Initialized") -> ("object out"=w255:refnum<class "Application.lvclass">)  [unwired: 16 in, 1 out]
      }
      frame "AD2MSOConfig" {
        n110 = call-dynamic "GetAD2_SDK.vi"("object in"=w272) -> ("object out"=w271:refnum<class "Application.lvclass">, "AD2_SDK"=w267:refnum<class "AD2_SDK.lvclass">)  [unwired: 16 in, 1 out]
        n111 = call-dynamic "ConfigMSO.vi"("object in"=w267, "variant"="MSO", "error in (no error)"=w268) -> ("object out"=w266:refnum<class "AD2_SDK.lvclass">, "error out"=w269:errorcluster)  [unwired: 15 in]
        n112 = call-dynamic "SetAD2_SDK.vi"("object in"=w271, "AD2_SDK"=w266) -> ("object out"=w270:refnum<class "Application.lvclass">)  [unwired: 16 in, 1 out]
        n113 = call-dynamic "FireUpdateStatus.vi"("object in"=w270, "Status"="MSO Configured") -> ("object out"=w264:refnum<class "Application.lvclass">)  [unwired: 16 in, 1 out]
      }
      frame "AD2MSORead" {
        n114 = call-dynamic "GetAD2_SDK.vi"("object in"=w282) -> ("object out"=w281:refnum<class "Application.lvclass">, "AD2_SDK"=w279:refnum<class "AD2_SDK.lvclass">)  [unwired: 16 in, 1 out]
        n115 = call-dynamic "ReadMSO.vi"("object in"=w279, "error in (no error)"=w277) -> ("object out"=w278:refnum<class "AD2_SDK.lvclass">, "Channels array"=→"Waveform Graph":waveform(dbl)[], "error out"=w276:errorcluster)  [unwired: 15 in]
        n116 = call-dynamic "SetAD2_SDK.vi"("object in"=w281, "AD2_SDK"=w278) -> ("object out"=w280:refnum<class "Application.lvclass">)  [unwired: 16 in, 1 out]
        n117 = call-dynamic "FireUpdateStatus.vi"("object in"=w280, "Status"="MSO Read") -> ("object out"=w275:refnum<class "Application.lvclass">)  [unwired: 16 in, 1 out]
      }
      frame "AD2Trigg" {
        n118 = call-dynamic "GetAD2_SDK.vi"("object in"=w291, "error in (no error)"=w287) -> ("object out"=w290:refnum<class "Application.lvclass">, "AD2_SDK"=w286:refnum<class "AD2_SDK.lvclass">, "error out"=w284:errorcluster)  [unwired: 15 in]
        n119 = call-dynamic "PCTrig.vi"("object in"=w286, "error in (no error)"=w284) -> ("object out"=w285:refnum<class "AD2_SDK.lvclass">, "error out"=w283:errorcluster)  [unwired: 16 in]
        n120 = call-dynamic "SetAD2_SDK.vi"("object in"=w290, "AD2_SDK"=w285, "error in (no error)"=w283) -> ("object out"=w289:refnum<class "Application.lvclass">, "error out"=w288:errorcluster)  [unwired: 15 in]
      }
      frame "PeltierInit" {
        n121 = call-dynamic "GetTC0608.vi"("object in"=w297) -> ("object out"=w299:refnum<class "Application.lvclass">, "TC0608"=w301:refnum<class "TC0608.lvclass">)  [unwired: 16 in, 1 out]
        n122 = call "TC0608_Init.vi"("object in"=w301, "VISA resource name"="Peltier VISA resource name", "error in (no error)"=w294) -> ("object out"=w300:refnum<class "TC0608.lvclass">, "error out"=w295:errorcluster)  [unwired: 15 in]
        n123 = call-dynamic "SetTC0608.vi"("object in"=w299, "TC0608"=w300) -> ("object out"=w298:refnum<class "Application.lvclass">)  [unwired: 16 in, 1 out]
        n124 = call-dynamic "UpdateStatus.vi"("object in"=w298, "Status"="Peltier Initialized") -> ("object out"=w293:refnum<class "Application.lvclass">)  [unwired: 16 in, 1 out]
      }
      frame "PeltierRead" {
        n125 = call-dynamic "GetTC0608.vi"("object in"=w307) -> ("object out"=w309:refnum<class "Application.lvclass">, "TC0608"=w306:refnum<class "TC0608.lvclass">)  [unwired: 16 in, 1 out]
        n126 = call-dynamic "ReadTemperature.vi"("object in"=w306, "error in (no error)"=w304) -> ("object out"=w305:refnum<class "TC0608.lvclass">, "temperature (C)"=→"temperature (C)":dbl, "error out"=w303:errorcluster)  [unwired: 15 in]
        n127 = call-dynamic "SetTC0608.vi"("object in"=w309, "TC0608"=w305) -> ("object out"=w308:refnum<class "Application.lvclass">)  [unwired: 16 in, 1 out]
      }
      frame "CetoniCheckLevelAndRefill" {
        n128 = call-dynamic "GetCetoniPump.vi"("object in"=w324, "error in (no error)"=w321) -> ("object out"=w310:refnum<class "Application.lvclass">, "CetoniPump"=w320:refnum<class "CetoniPump.lvclass">, "error out"=w312:errorcluster)  [unwired: 15 in]
        n129 = call-dynamic "ReadStatus.vi"("object in"=w320, "index"="index", "error in (no error)"=w312) -> ("object out"=w318:refnum<class "CetoniPump.lvclass">, "Fill Level"=w315:dbl, "error out"=w317:errorcluster)  [unwired: 12 in, 2 out]
        n130 = Less Or Equal?(x=w315, y="refill below level") -> (x <= y?=w316:bool)
        n131 = case shown="True" w316 {
          tunnel: "index" -> [_ w337]
          tunnel: w318 -> [w326 w333]
          tunnel: w317 -> [w325 w335]
          tunnel: [w326 w330] -> w313
          tunnel: [w325 w327] -> w311
          tunnel: w310 -> [_ w332]
          tunnel: w310 -> [_ w329]
          frame False {
          }
          frame True {
            n132 = call-dynamic "FireUpdateStatus.vi"("object in"=w332, "Status"="refilling") -> ()  [unwired: 16 in, 2 out]
            n133 = call-dynamic "Refill.vi"("object in"=w333, "index"=w337, "error in (no error)"=w335) -> ("object out"=w338:refnum<class "CetoniPump.lvclass">, "error out"=w336:errorcluster)  [unwired: 15 in]
            n134 = while {
              tunnel: w337 -> [w349]
              shift-right: [w339] -> w330
              shift-left: w338 -> [w350]
              shift-right: [w347] -> w327
              shift-left: w336 -> [w348]
              shift-right: [FALSE] -> _
              shift-left: TRUE -> [w341]
              stop <- w342 stop-if-true
              n135 = call-dynamic "ReadStatus.vi"("object in"=w350, "index"=w349, "error in (no error)"=w348) -> ("object out"=w339:refnum<class "CetoniPump.lvclass">, "Is pumping"=w345:bool, "error out"=w347:errorcluster)  [unwired: 12 in, 2 out]
              n136 = call "Elapsed Time"("Time Target (s)"="Timeout Refill", "Reset"=w341) -> ("Time has Elapsed"=w343:bool)  [unwired: 10 in, 7 out]
              n137 = Not(x=w345) -> (.not. x?=w344:bool)
              n138 = Or(x=w344, y=w343) -> (x .or. y?=w342:bool)
            }
            n139 = call-dynamic "FireUpdateStatus.vi"("object in"=w329, "Status"="refill complete", "error in (no error)"=w327) -> ()  [unwired: 15 in, 2 out]
          }
        }
        n140 = call-dynamic "SetCetoniPump.vi"("object in"=w310, "CetoniPump"=w313, "error in (no error)"=w311) -> ("object out"=w323:refnum<class "Application.lvclass">, "error out"=w322:errorcluster)  [unwired: 15 in]
      }
      frame "CetoniConfigureSyringe" {
        n141 = call-dynamic "GetCetoniPump.vi"("object in"=w361, "error in (no error)"=w357) -> ("object out"=w358:refnum<class "Application.lvclass">, "CetoniPump"=w356:refnum<class "CetoniPump.lvclass">, "error out"=w352:errorcluster)  [unwired: 15 in]
        n142 = call-dynamic "ConfigureSyringe.vi"("object in"=w356, "index"="index configure syringe", "SyringeSettings"="SyringeSettings", "error in (no error)"=w352) -> ("object out"=w355:refnum<class "CetoniPump.lvclass">, "error out"=w351:errorcluster)  [unwired: 14 in]
        n143 = call-dynamic "SetCetoniPump.vi"("object in"=w358, "CetoniPump"=w355, "error in (no error)"=w351) -> ("object out"=w360:refnum<class "Application.lvclass">, "error out"=w359:errorcluster)  [unwired: 15 in]
      }
      frame "CetoniEmpty" {
        n144 = Variant To Data(error in=w367, Variant=w369) -> (data=w362:i32, error out=w368:errorcluster)  [unwired: 1 in]
        n145 = call-dynamic "GetCetoniPump.vi"("object in"=w373, "error in (no error)"=w368) -> ("object out"=w370:refnum<class "Application.lvclass">, "CetoniPump"=w366:refnum<class "CetoniPump.lvclass">, "error out"=w364:errorcluster)  [unwired: 15 in]
        n146 = call-dynamic "Empty.vi"("object in"=w366, "index"=w362, "error in (no error)"=w364) -> ("object out"=w365:refnum<class "CetoniPump.lvclass">, "error out"=w363:errorcluster)  [unwired: 15 in]
        n147 = call-dynamic "SetCetoniPump.vi"("object in"=w370, "CetoniPump"=w365, "error in (no error)"=w363) -> ("object out"=w372:refnum<class "Application.lvclass">, "error out"=w371:errorcluster)  [unwired: 15 in]
      }
      frame "CetoniGoToLevel" {
        # "Updates Control with coerced\nvalues"
        n148 = local read "GoToLevelSettings"() -> (w377:T3)
        n149 = Variant To Data(error in=w378, type=w377, Variant=w380) -> (data=w376:T3, error out=w379:errorcluster)
        n150 = call-dynamic "GetCetoniPump.vi"("object in"=w389, "error in (no error)"=w379) -> ("object out"=w386:refnum<class "Application.lvclass">, "CetoniPump"=w383:refnum<class "CetoniPump.lvclass">, "error out"=w385:errorcluster)  [unwired: 15 in]
        n151 = call-dynamic "SetFillLevel.vi"("object in"=w383, "GoToLevelSettings"=w376, "error in (no error)"=w385) -> ("object out"=w382:refnum<class "CetoniPump.lvclass">, "Coerced Level"=w381:dbl, "Coerced Flow"=w375:dbl, "error out"=w384:errorcluster)  [unwired: 12 in, 1 out]
        n152 = Bundle By Name(cluster=w376, "Level(ml)"=w381, "Flow"=w375) -> (w374:T3)
        n153 = call-dynamic "SetCetoniPump.vi"("object in"=w386, "CetoniPump"=w382, "error in (no error)"=w384) -> ("object out"=w388:refnum<class "Application.lvclass">, "error out"=w387:errorcluster)  [unwired: 15 in]
        n154 = local write "GoToLevelSettings"(w374) -> ()
      }
      frame "CetoniInit" {
        n155 = call-dynamic "GetCetoniPump.vi"("object in"=w399, "error in (no error)"=w397) -> ("object out"=w395:refnum<class "Application.lvclass">, "CetoniPump"=w394:refnum<class "CetoniPump.lvclass">, "error out"=w392:errorcluster)  [unwired: 15 in]
        n156 = call "CetoniPump_Init.vi"("object in"=w394, "Device Configuration Path"="Device Configuration Folder", "error in (no error)"=w392) -> ("object out"=w393:refnum<class "CetoniPump.lvclass">, "error out"=w391:errorcluster)  [unwired: 15 in]
        n157 = call-dynamic "SetCetoniPump.vi"("object in"=w395, "CetoniPump"=w393, "error in (no error)"=w391) -> ("object out"=w398:refnum<class "Application.lvclass">, "error out"=w396:errorcluster)  [unwired: 15 in]
      }
      frame "CetoniReadStatus" {
        n158 = call-dynamic "GetCetoniPump.vi"("object in"=w412, "error in (no error)"=w409) -> ("object out"=w410:refnum<class "Application.lvclass">, "CetoniPump"=w408:refnum<class "CetoniPump.lvclass">, "error out"=w406:errorcluster)  [unwired: 15 in]
        n159 = call-dynamic "ReadStatusAllPumps.vi"("object in"=w408, "error in (no error)"=w406) -> ("object out"=w407:refnum<class "CetoniPump.lvclass">, "Array"=→"Pump Status":T1, "error out"=w405:errorcluster)  [unwired: 15 in]
        n160 = call-dynamic "SetCetoniPump.vi"("object in"=w410, "CetoniPump"=w407, "error in (no error)"=w405) -> ("object out"=w402:refnum<class "Application.lvclass">, "error out"=w411:errorcluster)  [unwired: 15 in]
        n161 = local read "Read Status"() -> (w400:bool)
        n162 = case shown="True" w400 {
          tunnel: "CetoniReadStatus" ("Message") -> [_ w416]
          tunnel: w402 -> [w413 w415]
          tunnel: [w413 w414] -> w401
          frame False {
          }
          frame True {
            n163 = call-dynamic "EnqueueMain.vi"("object in"=w415, "Message"=w416) -> ("object out"=w414:refnum<class "Application.lvclass">)  [unwired: 16 in, 1 out]
          }
        }
      }
      frame "CetoniReferenceMove" {
        n164 = call-dynamic "GetCetoniPump.vi"("object in"=w427, "error in (no error)"=w423) -> ("object out"=w424:refnum<class "Application.lvclass">, "CetoniPump"=w422:refnum<class "CetoniPump.lvclass">, "error out"=w419:errorcluster)  [unwired: 15 in]
        n165 = call-dynamic "GetConnectedPumps.vi"("object in"=w422) -> ("object out"=w421:refnum<class "CetoniPump.lvclass">, "ConnectedPumps"=w417:T17)  [unwired: 16 in, 1 out]
        n166 = for {
          shift-right: [w431] -> w420
          shift-left: w421 -> [w432]
          shift-right: [w429] -> w418
          shift-left: w419 -> [w430]
          tunnel: w417 -> [_] mode=indexing
          i -> [w428]
          n167 = call-dynamic "ReferenceMove.vi"("object in"=w432, "index"=w428, "error in (no error)"=w430) -> ("object out"=w431:refnum<class "CetoniPump.lvclass">, "error out"=w429:errorcluster)  [unwired: 15 in]
        }
        n168 = call-dynamic "SetCetoniPump.vi"("object in"=w424, "CetoniPump"=w420, "error in (no error)"=w418) -> ("object out"=w426:refnum<class "Application.lvclass">, "error out"=w425:errorcluster)  [unwired: 15 in]
      }
      frame "CetoniRefill" {
        n169 = Variant To Data(error in=w438, Variant=w440) -> (data=w433:i32, error out=w439:errorcluster)  [unwired: 1 in]
        n170 = call-dynamic "GetCetoniPump.vi"("object in"=w444, "error in (no error)"=w439) -> ("object out"=w441:refnum<class "Application.lvclass">, "CetoniPump"=w437:refnum<class "CetoniPump.lvclass">, "error out"=w435:errorcluster)  [unwired: 15 in]
        n171 = call-dynamic "Refill.vi"("object in"=w437, "index"=w433, "error in (no error)"=w435) -> ("object out"=w436:refnum<class "CetoniPump.lvclass">, "error out"=w434:errorcluster)  [unwired: 15 in]
        n172 = call-dynamic "SetCetoniPump.vi"("object in"=w441, "CetoniPump"=w436, "error in (no error)"=w434) -> ("object out"=w443:refnum<class "Application.lvclass">, "error out"=w442:errorcluster)  [unwired: 15 in]
      }
      frame "CetoniStopPumps" {
        n173 = call-dynamic "GetCetoniPump.vi"("object in"=w453, "error in (no error)"=w449) -> ("object out"=w450:refnum<class "Application.lvclass">, "CetoniPump"=w448:refnum<class "CetoniPump.lvclass">, "error out"=w446:errorcluster)  [unwired: 15 in]
        n174 = call-dynamic "StopAllPumps.vi"("object in"=w448, "error in (no error)"=w446) -> ("object out"=w447:refnum<class "CetoniPump.lvclass">, "error out"=w445:errorcluster)  [unwired: 16 in]
        n175 = call-dynamic "SetCetoniPump.vi"("object in"=w450, "CetoniPump"=w447, "error in (no error)"=w445) -> ("object out"=w452:refnum<class "Application.lvclass">, "error out"=w451:errorcluster)  [unwired: 15 in]
      }
      frame "ChangeFrequency" {
        n176 = Variant To Data(error in=w461, Variant=w463) -> (data=w458:dbl, error out=w462:errorcluster)  [unwired: 1 in]
        n177 = call-dynamic "GetAFG3022B.vi"("object in"=w464) -> ("object out"=w467:refnum<class "Application.lvclass">, "AFG3022B"=w466:refnum<class "AFG3022B.lvclass">)  [unwired: 16 in, 1 out]
        n178 = Wait (ms)(milliseconds to wait=u32 500) -> ()  [unwired: 1 out]
        n179 = call-dynamic "Frequency Change Channel 1.vi"("object in"=w466, "Frequency (1000 Hz)"=w458) -> ("object out"=w465:refnum<class "AFG3022B.lvclass">)  [unwired: 16 in, 1 out]
        n180 = Number To Fractional String(number=w458) -> (F-format string=w456:string)  [unwired: 3 in]
        n181 = Concatenate Strings("Changed Frequency: " ("Status"), w456) -> (w457:string)
        n182 = call-dynamic "SetAFG3022B.vi"("object in"=w467, "AFG3022B"=w465) -> ("object out"=w460:refnum<class "Application.lvclass">)  [unwired: 16 in, 1 out]
        n183 = call-dynamic "FireUpdateStatus.vi"("object in"=w460, "Status"=w457) -> ("object out"=w459:refnum<class "Application.lvclass">)  [unwired: 16 in, 1 out]
      }
      frame "ChangeVoltage" {
        n184 = Variant To Data(error in=w477, Variant=w479) -> (data=w469:dbl, error out=w478:errorcluster)  [unwired: 1 in]
        n185 = call-dynamic "GetAFG3022B.vi"("object in"=w480) -> ("object out"=w481:refnum<class "Application.lvclass">, "AFG3022B"=w470:refnum<class "AFG3022B.lvclass">)  [unwired: 16 in, 1 out]
        n186 = Wait (ms)(milliseconds to wait=u32 500) -> ()  [unwired: 1 out]
        n187 = call-dynamic "Change Voltage Channel 1.vi"("object in"=w470, "Amplitude (1 Vpp)"=w469) -> ("object out"=w471:refnum<class "AFG3022B.lvclass">)  [unwired: 16 in, 1 out]
        n188 = Number To Fractional String(number=w469) -> (F-format string=w473:string)  [unwired: 3 in]
        n189 = Concatenate Strings("Changed Voltage: " ("Status"), w473) -> (w474:string)
        n190 = call-dynamic "SetAFG3022B.vi"("object in"=w481, "AFG3022B"=w471) -> ("object out"=w476:refnum<class "Application.lvclass">)  [unwired: 16 in, 1 out]
        n191 = call-dynamic "FireUpdateStatus.vi"("object in"=w476, "Status"=w474) -> ("object out"=w475:refnum<class "Application.lvclass">)  [unwired: 16 in, 1 out]
      }
      frame "Error" {
        # "#CodeRecommended - If you ever change the name of this \"Error\" message, you'll need to update the name in the Check Loop Error.vi as well."
        # "#CodeRecommended - Consider creating a system for logging errors in some way. These errors are for notification purposes only. Handling of specific errors should be performed in the message frames that generated the error."
        # "Error - Display an error dialog. This message is sent by the \"Error Handler\" VIs at the end of other loops in this application."
        n192 = Variant To Data(error in=w488, type=errorcluster {"status"=FALSE, "code"=0, "source"=""} ("error constant"), Variant=w487) -> (data=w485:errorcluster, error out=w484:errorcluster)
        n193 = call <vilib>:"Simple Error Handler.vi"("error in (no error)"=w485) -> ()  [unwired: 4 in, 5 out]
        n194 = Merge Errors(w484) -> (w483:errorcluster)
      }
      frame "Exit" {
        # "Stop the VI"
        # "Release the message queue reference"
        # "#CodeNeeded - Add any required cleanup code here. Note that if 'Exit' was called as a result of an error, an error dialog will be displayed. Add any custom error handling for an 'Exit' condition here as well."
        # "Exit - Exit the application."
        n195 = call <vilib>:"Simple Error Handler.vi"("error in (no error)"=w490) -> ("error out"=w489:errorcluster)  [unwired: 4 in, 4 out]
        n196 = call-dynamic "FireStopEvent.vi"("object in"=w492, "error in (no error)"=w489) -> ("object out"=w493:refnum<class "Application.lvclass">, "error out"=w491:errorcluster)  [unwired: 16 in]
      }
      frame "FuncInit" {
        n197 = call-dynamic "GetAFG3022B.vi"("object in"=w500) -> ("object out"=w502:refnum<class "Application.lvclass">, "AFG3022B"=w499:refnum<class "AFG3022B.lvclass">)  [unwired: 16 in, 1 out]
        n198 = call "AFG3022B_Init.vi"("object in"=w499, "VISA resource name"="Function Generator", "error in (no error)"=w495) -> ("object out"=w498:refnum<class "AFG3022B.lvclass">, "error out"=w496:errorcluster)  [unwired: 15 in]
        n199 = call-dynamic "SetAFG3022B.vi"("object in"=w502, "AFG3022B"=w498) -> ("object out"=w501:refnum<class "Application.lvclass">)  [unwired: 16 in, 1 out]
      }
      frame "Initialize" {
        # "Initialize - All initialization work should take place in this message, since other loops can potentially enqueue messages that execute immediately after this one."
        n200 = Build Array("CoriolisInit", "CetoniInit", "HamamatsuInit", "AD2Init", "OscilloscopeInit" ("element"), "PeltierInit" ("element")) -> (w510:string[])
        n201 = for {
          shift-right: [w514] -> w508
          shift-left: w507 -> [w515]
          tunnel: w510 -> [w513] mode=indexing
          n202 = call-dynamic "EnqueueMain.vi"("object in"=w515, "Message"=w513) -> ("object out"=w514:refnum<class "Application.lvclass">)  [unwired: 16 in, 1 out]
        }
      }
      frame "InjectError" {
        # "Something Else - Replace this message with functionality for your own application."
        n203 = Variant To Data(error in=w517, type=errorcluster {"status"=FALSE, "code"=0, "source"=""} ("error in (no error)"), Variant=w520) -> (data=w516:errorcluster, error out=w518:errorcluster)
        n204 = Merge Errors(w516, w518) -> (w522:errorcluster)
      }
      frame "OscilloscopeInit" {
        n205 = call-dynamic "GetTBS2000.vi"("object in"=w526) -> ("object out"=w524:refnum<class "Application.lvclass">, "TBS2000Series"=w527:refnum<class "TBS2000Series.lvclass">)  [unwired: 16 in, 1 out]
        n206 = call "TBS2000Series_Init.vi"("object in"=w527, "VISA resource name"="Oscilloscope", "error in (no error)"=w529) -> ("object out"=w523:refnum<class "TBS2000Series.lvclass">, "error out"=w528:errorcluster)  [unwired: 15 in]
        n207 = call-dynamic "Set TBS2000.vi"("object in"=w524, "TBS2000Series"=w523) -> ("object out"=w525:refnum<class "Application.lvclass">)  [unwired: 16 in, 1 out]
      }
      frame "ReadOscilloscope" {
        # "Have options to read any singular value from the oscilloscope. Also display waveform for a channel the user picks."
      }
      frame "ReadTemperature" {
        # "Read the Temperature and write into textfile"
      }
      frame "SaveDataEacExperiment" {
        n208 = call-dynamic "GetTC0608.vi"("object in"=w558) -> ("object out"=w557:refnum<class "Application.lvclass">, "TC0608"=w556:refnum<class "TC0608.lvclass">)  [unwired: 16 in, 1 out]
        n209 = call-dynamic "ReadTemperature.vi"("object in"=w556, "error in (no error)"=w554) -> ("object out"=w555:refnum<class "TC0608.lvclass">, "temperature (C)"=w541:dbl, "error out"=w543:errorcluster)  [unwired: 15 in]
        "Temperatur (C)" <- w541
        n210 = call-dynamic "SetTC0608.vi"("object in"=w557, "TC0608"=w555) -> ("object out"=w552:refnum<class "Application.lvclass">)  [unwired: 16 in, 1 out]
        n211 = call-dynamic "GetTBS2000.vi"("object in"=w552) -> ("object out"=w553:refnum<class "Application.lvclass">, "TBS2000Series"=w551:refnum<class "TBS2000Series.lvclass">)  [unwired: 16 in, 1 out]
        n212 = Variant To Data(type=T10 {"Frequencies (MHz)"=[], "Camera Settings"={"Minimum Time between\n frames(s)"=10.0, "Number of Frames"=0}, "Flowrates (ul/min)"=[], "Voltages (V)"=[]} ("Experiment Settings"), Variant=w540) -> (data=w538:T10)  [unwired: 1 in, 1 out]
        n213 = call-dynamic "Read Osc. Energy Density.vi"("object in"=w551, "Oscilloscope"="Oscilloscope", "error in (no error)"=w543) -> ("object out"=w550:refnum<class "TBS2000Series.lvclass">, "Oscilloscope\n Results"=w537:T11, "error out"=w544:errorcluster)  [unwired: 10 in]
        "Oscilloscope Results" <- w537
        n214 = call-dynamic "Set TBS2000.vi"("object in"=w553, "TBS2000Series"=w550) -> ("object out"=w535:refnum<class "Application.lvclass">)  [unwired: 16 in, 1 out]
        n215 = call-dynamic "GetSaveData.vi"("object in"=w535) -> ("object out"=w548:refnum<class "Application.lvclass">, "SaveData"=w547:refnum<class "SaveData.lvclass">)  [unwired: 16 in, 1 out]
        n216 = call "EacExperiment.vi"("object in"=w547, "Path"="SaveFolder", "Temperature (C)"=w541, "Oscilloscope Results"=w537, "Experiment Settings"=w538, "error in (no error)"=w544) -> ("object out"=w546:refnum<class "SaveData.lvclass">, "error out"=w542:errorcluster)  [unwired: 12 in]
        n217 = call-dynamic "SetSaveData.vi"("object in"=w548, "SaveData"=w546) -> ("object out"=w545:refnum<class "Application.lvclass">)  [unwired: 16 in, 1 out]
      }
      frame "Something" {
        # "Send string to \"Update Display\" message"
        # "#CodeNeeded - Perform whatever actions correspond to the \"Something\" message."
        # "Something - Replace this message with functionality for your own application."
        n218 = Merge Errors(w560) -> (w561:errorcluster)
      }
      frame "TakeNImages" {
        # "This Constants is set to give a 1ms pulse over 5ms span, pc triggered, and then wait for new trigger\nDo not Change unless you know how to set the DOs of the AD2"
        n219 = Variant To Data(error in=w565, type=T16 {"Minimum Time between frames"=10.0, "Number of Frames"=0} ("Image  Aquisition"), Variant=w568) -> (data=w564:T16, error out=w566:errorcluster)
        n220 = Unbundle By Name(w564) -> ("Number of Frames"=w563:i32, "Minimum Time between frames"=w562:dbl)
        n221 = call-dynamic "GetAD2_SDK.vi"("object in"=w572) -> ("object out"=w571:refnum<class "Application.lvclass">, "AD2_SDK"=w577:refnum<class "AD2_SDK.lvclass">, "error out"=w576:errorcluster)  [unwired: 16 in]
        n222 = call-dynamic "ConfigDO.vi"("object in"=w577, 2:T12 {"DO Trigger"={"secRun(0=Cont)"=0.005, "secWait"=0.0, "cRepeat(0=inf)"=0, "Repeat Trigger"=TRUE, "TrigrSrc"=enum."trigsrcPC"}, "CustomData"=[{"Data"=[FALSE, TRUE, FALSE, FALSE, FALSE, FALSE, FALSE, FALSE, FALSE, FALSE, FALSE, FALSE, FALSE, FALSE, FALSE, FALSE, FALSE, FALSE, FALSE, FALSE, FALSE, FALSE], "Freq"=1000.0, "#Bits"=100, "Enable"=TRUE, "IdleState"=0}, {"Data"=[], "Freq"=0.0, "#Bits"=0, "Enable"=FALSE, "IdleState"=0}, {"Data"=[], "Freq"=0.0, "#Bits"=0, "Enable"=FALSE, "IdleState"=0}, {"Data"=[], "Freq"=0.0, "#Bits"=0, "Enable"=FALSE, "IdleState"=0}, {"Data"=[], "Freq"=0.0, "#Bits"=0, "Enable"=FALSE, "IdleState"=0}, {"Data"=[], "Freq"=0.0, "#Bits"=0, "Enable"=FALSE, "IdleState"=0}, {"Data"=[], "Freq"=0.0, "#Bits"=0, "Enable"=FALSE, "IdleState"=0}, {"Data"=[], "Freq"=0.0, "#Bits"=0, "Enable"=FALSE, "IdleState"=0}, {"Data"=[], "Freq"=0.0, "#Bits"=0, "Enable"=FALSE, "IdleState"=0}, {"Data"=[], "Freq"=0.0, "#Bits"=0, "Enable"=FALSE, "IdleState"=0}, {"Data"=[], "Freq"=0.0, "#Bits"=0, "Enable"=FALSE, "IdleState"=0}, {"Data"=[], "Freq"=0.0, "#Bits"=0, "Enable"=FALSE, "IdleState"=0}, {"Data"=[], "Freq"=0.0, "#Bits"=0, "Enable"=FALSE, "IdleState"=0}]}, "error in (no error)"=w576) -> ("object out"=w574:refnum<class "AD2_SDK.lvclass">, "error out"=w575:errorcluster)  [unwired: 15 in]
        n223 = for {
          N: w563 -> [_]
          shift-right: [w582] -> w578
          shift-left: w575 -> [w587]
          shift-right: [w588] -> w579
          shift-left: w574 -> [w586]
          shift-right: [w584] -> w570
          shift-left: w571 -> [w585]
          tunnel: w562 -> [w580]
          stop <- w581 stop-if-true
          n224 = call-dynamic "PCTrig.vi"("object in"=w586, "error in (no error)"=w587) -> ("object out"=w588:refnum<class "AD2_SDK.lvclass">, "error out"=w583:errorcluster)  [unwired: 16 in]
          n225 = call-dynamic "Wait.vi"("object in"=w585, "Time to wait"=w580, "error in (no error)"=w583) -> ("object out"=w584:refnum<class "Application.lvclass">, "aborted"=w581:bool, "error out"=w582:errorcluster)  [unwired: 14 in]
        }
        n226 = call-dynamic "SetAD2_SDK.vi"("object in"=w570, "AD2_SDK"=w579, "error in (no error)"=w578) -> ("object out"=w573:refnum<class "Application.lvclass">)  [unwired: 15 in, 1 out]
      }
      frame "Wait" {
        n227 = Variant To Data(error in=w597, Variant=w599) -> (data=w598:dbl, error out=w594:errorcluster)  [unwired: 1 in]
        n228 = call-dynamic "FireUpdateStatus.vi"("object in"=w595, "Status"="waiting.....") -> ("object out"=w592:refnum<class "Application.lvclass">)  [unwired: 16 in, 1 out]
        n229 = call-dynamic "Wait.vi"("object in"=w592, "Time to wait"=w598, "error in (no error)"=w594) -> ("object out"=w596:refnum<class "Application.lvclass">, "error out"=w593:errorcluster)  [unwired: 14 in, 1 out]
        n230 = call-dynamic "FireUpdateStatus.vi"("object in"=w596, "Status"="wait complete") -> ("object out"=w590:refnum<class "Application.lvclass">)  [unwired: 16 in, 1 out]
      }
      frame Default {
        # "'Default' case only runs if there is a message that isn't defined in any of the other cases.  Output a programming error."
        n231 = xnode "Error Ring"("parameter 0"=w601) -> ("error out"=w602:errorcluster)
      }
    }
    n232 = call-dynamic "ErrorHandlerMainLoop.vi"("object in"=w226, "error in (no error)"=w229) -> ("object out"=w227:refnum<class "Application.lvclass">, "error out"=w228:errorcluster)  [unwired: 16 in]
  }
  n233 = Merge Errors(w5, w6) -> (w4:errorcluster)
  n234 = call-dynamic "CleanUp.vi"("object in"=w7, "error in (no error)"=w4) -> ("error out"=→"error out":errorcluster)  [unwired: 16 in, 1 out]
